vi "sub-dir-2.vi"() -> ()   [LabVIEW 2017]
panel:
  out "Numeric 2":i32
  in  "Numeric":i32
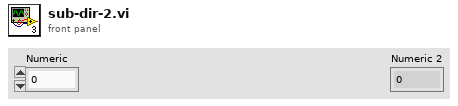
[diagram p1: front panel]
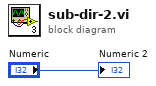
[diagram p0: block diagram]
diagram:
  "Numeric 2" <- "Numeric"
